vi "FZ_map.vi"(9 "Fz":dbl[][][](array[numeric]), 11 "Position":dbl[](array[numeric])) -> (1 "Rot(theta)":dbl[][](array[numeric]) format="%_3g", 3 "FZ-mapped":dbl[][][](array[numeric]))   [LabVIEW 2019]
uses:
  <vilib>/Analysis/baseanly.llb/Real A x B.vi
  <vilib>/Analysis/NI_AALBase.lvlib
panel:
  # "x\n\ny\n\ntheta"
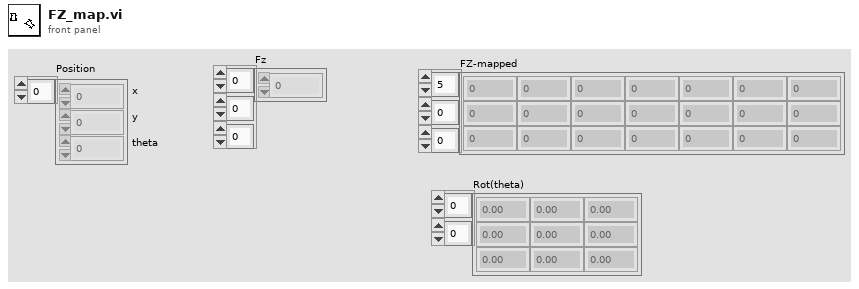
[diagram p1: front panel]
types:
  T1 = typedef "NI_Matrix.lvlib/RealMatrix.ctl" = dbl[][]
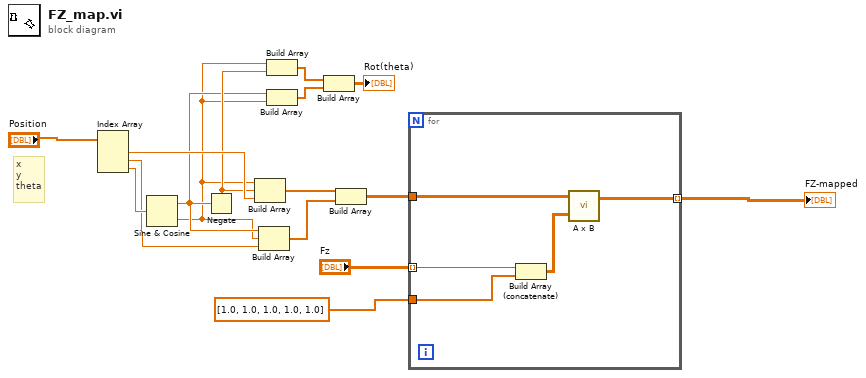
[diagram p0: block diagram]
diagram:
  # "x\ny\ntheta"
  n1 = Index Array(array="Position") -> (element #1=w14:dbl, element #2=w13:dbl, element #3=w15:dbl)  [unwired: 3 in]
  n2 = Sine & Cosine(0:w15) -> (1:w5:dbl, 2:w4:dbl)
  n3 = Negate(x=w5) -> (-x=w6:dbl)
  n4 = Build Array(w4, w6, w14) -> (w12:dbl[])
  n5 = Build Array(w5, w4, w13) -> (w11:dbl[])
  n6 = Build Array(w4, w6) -> (w3:dbl[])
  n7 = Build Array(w5, w4) -> (w2:dbl[])
  n8 = Build Array(w3, w2) -> (→"Rot(theta)":dbl[][])
  n9 = Build Array(w12, w11) -> (w8:dbl[][])
  n10 = for {
    tunnel: "Fz" -> [w21] mode=indexing
    tunnel: dbl[] [1.0, 1.0, 1.0, 1.0, 1.0] -> [w20]
    tunnel: w8 -> [w19]
    tunnel: [w17] -> w7 mode=indexing
    n11 = Build Array (concatenate)(w21, w20) -> (w18:dbl[][])
    n12 = call-poly <vilib>:"A x B.vi"("B"=w18, "A"=w19) -> ("A x B"=w17:T1)  [unwired: 1 out]
  }
  "FZ-mapped" <- w7
